vi "Start Audio FIFOs.vi"(8 "Error In":errorcluster, 11 "Audio Analyzer In":refnum<class "Audio Analyzer.lvclass">) -> (0 "Error Out":errorcluster, 3 "Audio Analyzer Out":refnum<class "Audio Analyzer.lvclass">)   [LabVIEW 2019, in "Audio Analyzer.lvclass"]
uses:
  Audio Analyzer.lvclass
  Accessors/FPGA Reference/Get FPGA Reference.vi
  <vilib>/Utility/error.llb/Error Cluster From Error Code.vi
  Public/Controls/FPGA Reference.ctl
  <vilib>/rvi/interface/nirviMethod/nirviMethod.xnode
  <vilib>/rvi/errors/niLvFpgaMergeErrorWithErrorCode.vi
  <vilib>/FPGAPlugInAG/Dynamic/niLvFpga_StartFifo_Dynamic.vi
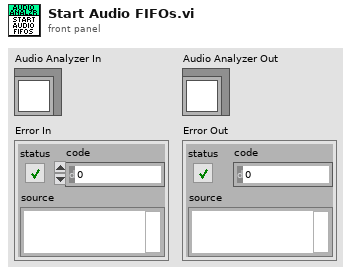
[diagram p1: front panel]
types:
  T1 = typedef "Audio Analyzer.lvclass/FPGA Reference.ctl" = refnum<k20>
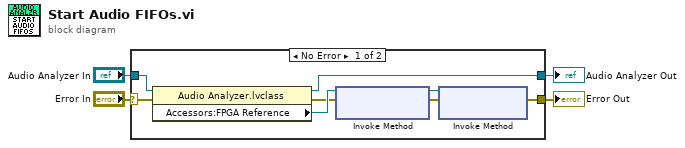
[diagram p0: block diagram]
diagram:
  n1 = case shown="No Error" "Error In" {
    selector: "Error In" -> [w10 w13]
    tunnel: [w5 w13] -> w4
    tunnel: "Audio Analyzer In" -> [w9 w14]
    tunnel: [w6 w14] -> w1
    frame No Error {
      n2 = property class="Audio Analyzer.lvclass"(reference=w9, error in=w10) -> (reference out=w6:refnum<class "Audio Analyzer.lvclass">, error out=w7:errorcluster, "Accessors:FPGA Reference"=w8:T1)
      n3 = xnode "Invoke Method"("FPGA VI Reference In"=w8, "error in"=w7) -> ("FPGA VI Reference Out"=w11:T1, "error out"=w12:errorcluster)
      n4 = xnode "Invoke Method"("FPGA VI Reference In"=w11, "error in"=w12) -> ("error out"=w5:errorcluster)  [unwired: 1 out]
    }
    frame Error {
    }
  }
  "Error Out" <- w4
  "Audio Analyzer Out" <- w1
